vi "Engaging.vi"(6 "PID Cluster":T2={"L1 to L4 PID Cluster"={"L1 PID Gains"={"Kp"=0.005, "Kd"=0.5, "Ki"=0.0005}, "L2 PID Gains"={"Kp"=0.01, "Kd"=1.0, "Ki"=0.005}, "L3 PID Gains"={"Kp"=0.05, "Kd"=1.0, "Ki"=0.0005}, "L4 PID Gains"={"Kp"=0.1, "Kd"=0.1, "Ki"=0.0005}}, "Stage PID Cluster"={"Stage Z PID"={"Kp"=0.0005, "Kd"=0.001, "Ki"=0.0}, "Stage Y PID"={"Kp"=0.0003, "Kd"=0.01, "Ki"=0.0}, "Stage X PID"={"Kp"=0.0003, "Kd"=0.01, "Ki"=0.0}}, "OCT Z PID Gains"={"Kp"=0.0003, "Kd"=0.0001, "Ki"=0.01}}, 7 "Offset Home 2 RCM":dbl[](array[numeric])=[0.0, 0.0, 0.0, 0.0], 8 "error in":errorcluster, 9 "Engage Pt":dbl[](array[numeric])=[0.0, 0.0, 0.0, 0.0], 10 "Prev Posit Cluster":T3={"Prev L1 to L4 Posit"=[0.0, 0.0, 0.0, 0.0], "Prev Stage Posit"=[6.0, 6.0, 6.0], "Prev OCT Z Posit"=0.0}, 11 "FPGA VI Reference In":refnum<k20>) -> (0 "error out":errorcluster, 2 "Last Posit Cluster":T1={"Last L1 to L4 Posit"=[0.0, 0.0, 0.0, 0.0], "Last Stage Posit"=[6.0, 6.0, 6.0], "Last OCT Z Posit"=0.0}, 3 "FPGA VI Reference Out":refnum<k20>)   [LabVIEW 2016]
uses:
  Global Variables.vi
  <vilib>/Platform/TimedLoop/XDataNode/wakeup.ctl
  <vilib>/Platform/TimedLoop/XDataNode/XDNodeRunTimeDep.lvlib
  <vilib>/Platform/TimedLoop/XDataNode/nitl_modes.ctl
  <vilib>/Platform/TimedLoop/XDataNode/timing_clust.ctl
  <vilib>/platform/TimedLoop/XDataNode/XDataNode.xnode
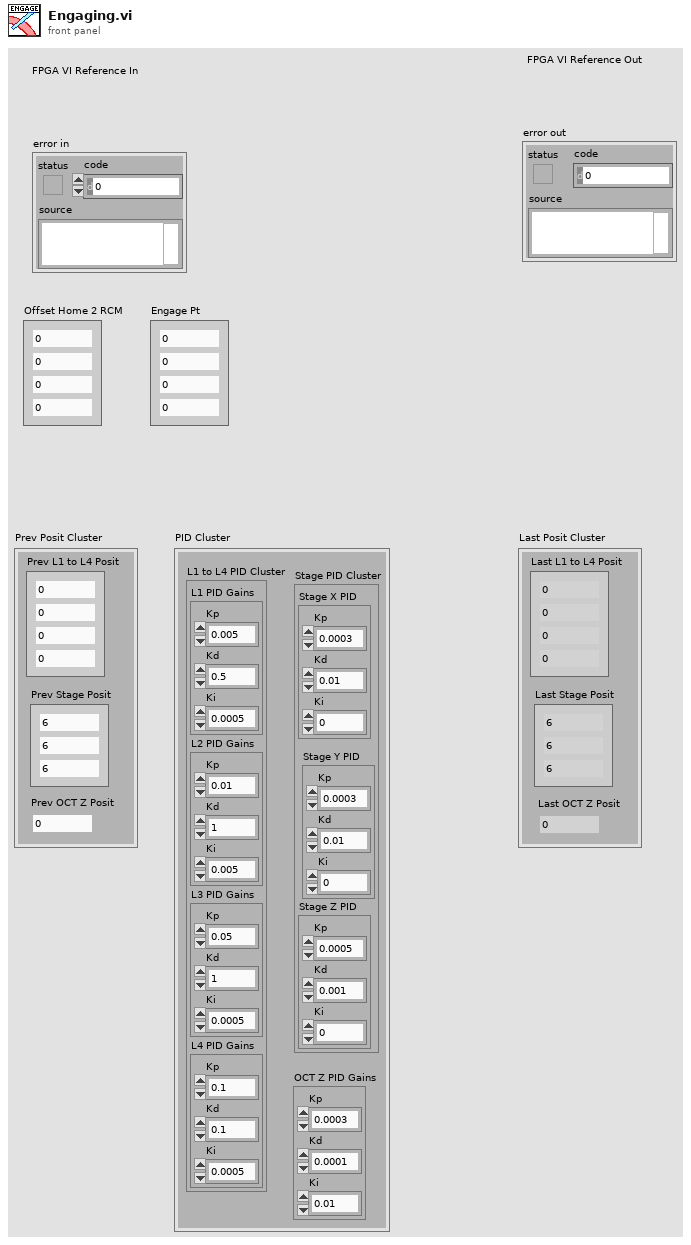
[diagram p1: front panel]
types:
  T1 = cluster{"Last L1 to L4 Posit":dbl[], "Last Stage Posit":dbl[], "Last OCT Z Posit":dbl}
  T2 = cluster{"L1 to L4 PID Cluster":cluster{"L1 PID Gains":cluster{"Kp":dbl, "Kd":dbl, "Ki":dbl}, "L2 PID Gains":cluster{"Kp":dbl, "Kd":dbl, "Ki":dbl}, "L3 PID Gains":cluster{"Kp":dbl, "Kd":dbl, "Ki":dbl}, "L4 PID Gains":cluster{"Kp":dbl, "Kd":dbl, "Ki":dbl}}, "Stage PID Cluster":cluster{"Stage Z PID":cluster{"Kp":dbl, "Kd":dbl, "Ki":dbl}, "Stage Y PID":cluster{"Kp":dbl, "Kd":dbl, "Ki":dbl}, "Stage X PID":cluster{"Kp":dbl, "Kd":dbl, "Ki":dbl}}, "OCT Z PID Gains":cluster{"Kp":dbl, "Kd":dbl, "Ki":dbl}}
  T3 = cluster{"Prev L1 to L4 Posit":dbl[], "Prev Stage Posit":dbl[], "Prev OCT Z Posit":dbl}
  T4 = typedef "XDNodeRunTimeDep.lvlib/timing_clust.ctl" = cluster{"Expected End [f-1]":u64, "Actual End [f-1]":u64, "Finished Late? [f-1]":bool, "Expected End [i-1]":u64, "Actual End [i-1]":u64, "Finished Late? [i-1]":bool, "Expected Start [i]":u64, "Actual Start [i]":u64, "Expected Start [f]":u64, "Actual Start [f]":u64, "Source Name":string, "Structure Name":string, "Period":i64, "Deadline":i64, "Offset":i64, "Start":i64, "Priority":i32, "Timeout":i32, "Mode":T5, "Wakeup Reason":T6, "Error":errorcluster, "Source Type":string, "Secondary Source Type":string, "Global End Time":u64, "Global Start Time":u64, "Frame Duration":u64, "Iteration Duration":u64, "Assigned CPU":i32, "I/O Scan Engine Mode":u32}
  T5 = typedef "XDNodeRunTimeDep.lvlib/nitl_modes.ctl" = enum32{"No Change", "Process missed periods, maintain original phase", "Discard missed periods, maintain original phase", "Process missed periods, ignore original phase", "Discard missed periods, ignore original phase"}
  T6 = typedef "XDNodeRunTimeDep.lvlib/wakeup.ctl" = enum32{"Normal", "Aborted", "Asynchronous wakeup", "Timing source error", "Timed loop error", "Timeout"}
  T7 = cluster{"Stage Z PID":cluster{"Kp":dbl, "Kd":dbl, "Ki":dbl}, "Stage Y PID":cluster{"Kp":dbl, "Kd":dbl, "Ki":dbl}, "Stage X PID":cluster{"Kp":dbl, "Kd":dbl, "Ki":dbl}}
  T8 = cluster{"L1 PID Gains":cluster{"Kp":dbl, "Kd":dbl, "Ki":dbl}, "L2 PID Gains":cluster{"Kp":dbl, "Kd":dbl, "Ki":dbl}, "L3 PID Gains":cluster{"Kp":dbl, "Kd":dbl, "Ki":dbl}, "L4 PID Gains":cluster{"Kp":dbl, "Kd":dbl, "Ki":dbl}}
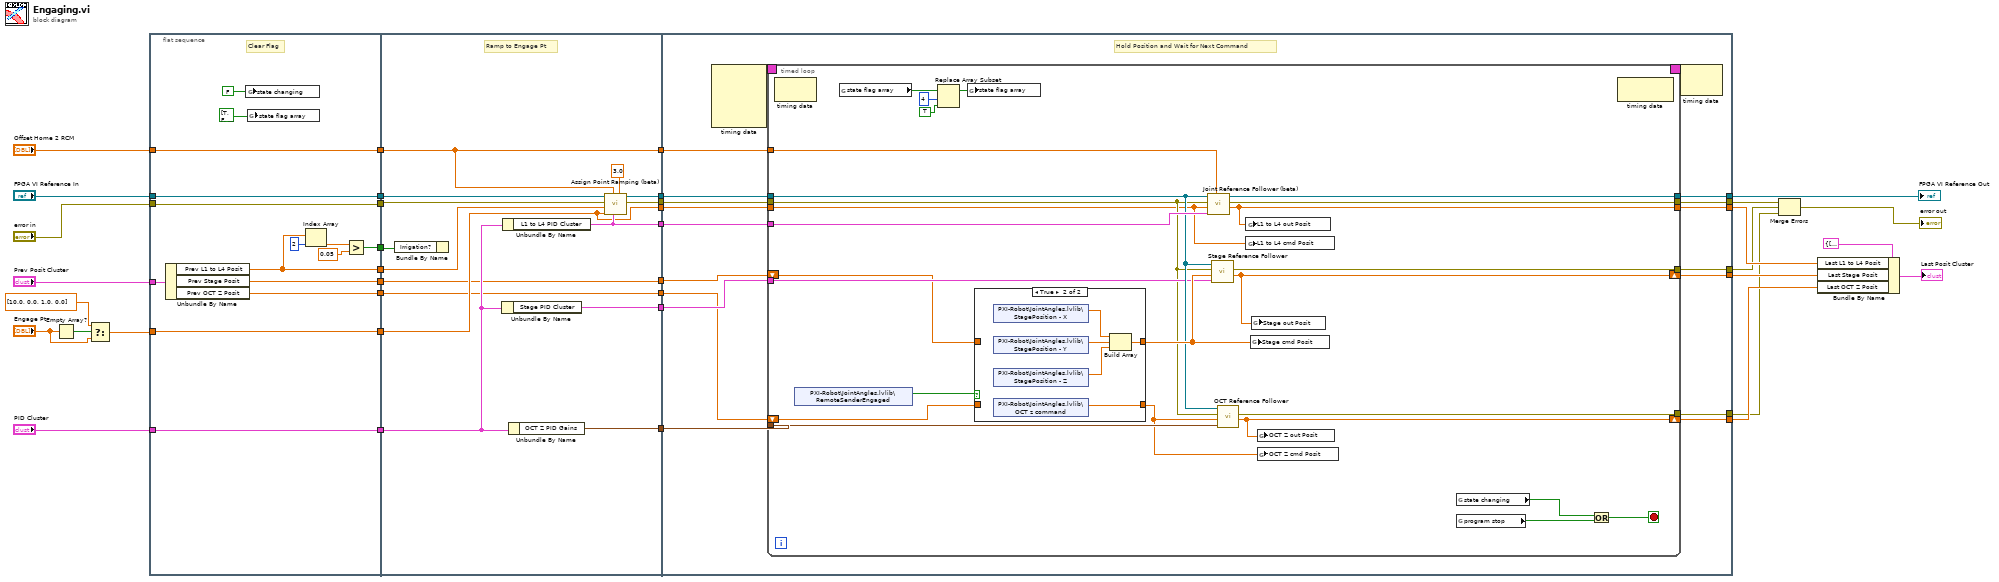
[diagram p0: block diagram]
diagram:
  n1 = Empty Array?(array="Engage Pt") -> (empty?=w29:bool)
  n2 = Select(t=dbl[] [10.0, 0.0, 1.0, 0.0] ("First Trk Pt 2"), s=w29, f="Engage Pt") -> (s? t:f=w26:dbl[])
  n3 = flat-sequence {
    tunnel: [w50] -> w37
    tunnel: "FPGA VI Reference In" -> [w50]
    tunnel: "error in" -> [w49]
    tunnel: [w49] -> w36
    tunnel: [w39] -> w35
    tunnel: "PID Cluster" -> [w47]
    tunnel: "Offset Home 2 RCM" -> [w48]
    tunnel: [w48] -> w33
    tunnel: [w43] -> w31
    tunnel: w26 -> [w43]
    tunnel: [w47] -> w19
    tunnel: "Prev Posit Cluster" -> [w46]
    tunnel: [w45] -> w5
    tunnel: [w44] -> w2
    tunnel: [w38] -> w1
    tunnel: w37 -> [w67]
    tunnel: w36 -> [w66]
    tunnel: w35 -> [w64]
    tunnel: w33 -> [w61]
    tunnel: w31 -> [w56]
    tunnel: [w63] -> w30
    tunnel: [w56] -> w25
    tunnel: [w62] -> w24
    tunnel: [w61] -> w23
    tunnel: [w60] -> w22
    tunnel: w19 -> [w58]
    tunnel: [w59] -> w18
    tunnel: [w57] -> w17
    tunnel: w5 -> [w55]
    tunnel: [w55] -> w4
    tunnel: [w54] -> w3
    tunnel: w2 -> [w54]
    tunnel: w1 -> [w53]
    tunnel: [w79] -> w13
    tunnel: [w78] -> w8
    tunnel: w30 -> [w82]
    tunnel: w25 -> [w81]
    tunnel: w24 -> [w83]
    tunnel: w23 -> [w70]
    tunnel: w22 -> [w80]
    tunnel: [w77] -> w20
    tunnel: [w76] -> w21
    tunnel: w18 -> [w75]
    tunnel: w17 -> [w74]
    tunnel: [w73] -> w14
    tunnel: [w72] -> w7
    tunnel: [w71] -> w6
    tunnel: w4 -> [w69]
    tunnel: w3 -> [w68]
    frame #0 {
      # "Clear Flag"
      n4 = Unbundle By Name(w46) -> ("Prev L1 to L4 Posit"=w39:dbl[], "Prev Stage Posit"=w45:dbl[], "Prev OCT Z Posit"=w44:dbl)
      n5 = global write "Global Variables.vi" "state changing"(FALSE ("state changing")) -> ()
      n6 = global write "Global Variables.vi" "state flag array"(bool[] [TRUE, FALSE, FALSE, FALSE, FALSE, FALSE, FALSE, FALSE, FALSE] ("state flag array")) -> ()
      n7 = Index Array(array=w39, index=2) -> (element=w41:dbl)
      n8 = Greater?(x=w41, y=0.05) -> (0:w38:bool)
    }
    frame #1 {
      # "Ramp to Engage Pt"
      n9 = Bundle By Name("Irrigation?"=w53) -> ()  [unwired: 1 in, 1 out]
      n10 = Unbundle By Name(w58) -> ("Stage PID Cluster"=w59:T7)
      n11 = Unbundle By Name(w58) -> ("L1 to L4 PID Cluster"=w60:T8)
      n12 = Unbundle By Name(w58) -> ("OCT Z PID Gains"=w57:cluster{"Kp":dbl, "Kd":dbl, "Ki":dbl})
      n13 = call "Assign Point Ramping (beta).vi"("Ramp Time [sec]"=3.0, "L1 to L4 PID Cluster"=w60, "Offset Home2RCM"=w61, "Destination Posit Array [mm]"=w56, "Previous Posit Array"=w64, "error in"=w66, "FPGA VI Reference In"=w67) -> ("error out"=w63:errorcluster, "FPGA VI Reference Out"=w62:refnum<k20>)  [unwired: 2 in, 1 out]
    }
    frame #2 {
      # "Hold Position and Wait for Next Command"
      n14 = node-c288() -> (w85:T4)  [unwired: 4 in]
      n15 = timed-loop {
        timing: w85 -> [_]
        timing-out: [_] -> w84
        tunnel: w83 -> [w100]
        tunnel: w82 -> [w92]
        tunnel: w70 -> [w106]
        tunnel: w81 -> [w86]
        tunnel: w80 -> [w105]
        tunnel: [w104] -> w79
        tunnel: [w103] -> w78
        tunnel: [w98] -> w77
        tunnel: w75 -> [w97]
        tunnel: w74 -> [w96]
        tunnel: [w91] -> w72
        tunnel: [w90] -> w71
        shift-right: [w101] -> w76
        shift-left: w69 -> [w88]
        shift-right: [w95] -> w73
        shift-left: w68 -> [w87]
        stop <- w93 stop-if-true
        n16 = node-c288() -> ()  [unwired: 1 in, 1 out]
        n17 = shared-variable "PXI-Robot\\JointAngles.lvlib\\RemoteSenderEngaged"() -> (w89:bool)  [unwired: 1 in, 1 out]
        n18 = global read "Global Variables.vi" "state flag array"() -> (w110:bool[])
        n19 = Replace Array Subset(array=w110, new element=TRUE ("new element/subarray"), index=4) -> (w109:bool[])
        n20 = global write "Global Variables.vi" "state flag array"(w109) -> ()
        n21 = case shown="True" w89 {
          tunnel: [w113 w115] -> w102
          tunnel: [w112 w114] -> w94
          tunnel: w88 -> [w113 _]
          tunnel: w87 -> [w112 _]
          frame False {
            # "Hold Position if not Engaged"
          }
          frame True {
            n22 = shared-variable "PXI-Robot\\JointAngles.lvlib\\StagePosition - X"() -> (w118:dbl)  [unwired: 1 in, 1 out]
            n23 = shared-variable "PXI-Robot\\JointAngles.lvlib\\StagePosition - Y"() -> (w117:dbl)  [unwired: 1 in, 1 out]
            n24 = shared-variable "PXI-Robot\\JointAngles.lvlib\\StagePosition - Z"() -> (w116:dbl)  [unwired: 1 in, 1 out]
            n25 = shared-variable "PXI-Robot\\JointAngles.lvlib\\OCT z command"() -> (w114:dbl)  [unwired: 1 in, 1 out]
            n26 = Build Array(w118, w117, w116) -> (w115:dbl[])
          }
        }
        n27 = call "Joint Reference Follower (beta).vi"("Offset Home2RCM [deg/mm]"=w106, "PID Ctrl Cluster"=w105, "Ref Array [deg/mm]"=w86, "error in"=w92, "FPGA VI Reference In"=w100) -> ("Output Posit Array [deg/mm]"=w98:dbl[], "error out"=w103:errorcluster, "FPGA VI Reference Out"=w104:refnum<k20>)  [unwired: 4 in]
        n28 = call "Stage Reference Follower.vi"("Stage PID Cluster"=w97, "Stage cmd Posit [mm]"=w102, "error in"=w92, "FPGA VI Reference In"=w100) -> ("Stage out Posit [mm]"=w101:dbl[], "error out"=w91:errorcluster)  [unwired: 5 in, 1 out]
        n29 = call "OCT Reference Follower.vi"("OCT Z PID Gains"=w96, "OCT  Z cmd Posit [mm]"=w94, "error in"=w92, "FPGA VI Reference In"=w100) -> ("OCT  Z out Posit [mm]"=w95:dbl, "error out"=w90:errorcluster)  [unwired: 5 in, 1 out]
        n30 = global write "Global Variables.vi" "L1 to L4 out Posit"(w98) -> ()
        n31 = global write "Global Variables.vi" "L1 to L4 cmd Posit"(w86) -> ()
        n32 = global write "Global Variables.vi" "Stage cmd Posit"(w102) -> ()
        n33 = global write "Global Variables.vi" "Stage out Posit"(w101) -> ()
        n34 = global write "Global Variables.vi" "OCT Z out Posit"(w95) -> ()
        n35 = global write "Global Variables.vi" "OCT Z cmd Posit"(w94) -> ()
        n36 = global read "Global Variables.vi" "state changing"() -> (w111:bool)
        n37 = global read "Global Variables.vi" "program stop"() -> (w99:bool)
        n38 = Or(x=w111, y=w99) -> (x .or. y?=w93:bool)
        n39 = node-c288() -> ()  [unwired: 1 in, 1 out]
      }
      n40 = node-c288(w84) -> ()  [unwired: 1 out]
    }
  }
  n41 = Merge Errors(w8, w7, w6) -> (→"error out":errorcluster)
  n42 = Bundle By Name(cluster=T1 {"Last L1 to L4 Posit"=[0.0, 0.0, 0.0, 0.0], "Last Stage Posit"=[6.0, 6.0, 6.0], "Last OCT Z Posit"=0.0} ("Last Posit Cluster 2"), "Last L1 to L4 Posit"=w20, "Last Stage Posit"=w21, "Last OCT Z Posit"=w14) -> (→"Last Posit Cluster":T1)
  "FPGA VI Reference Out" <- w13
